vi "CTRE_Phoenix_CANifier_SetControlFramePeriod.vi"(8 "error in (no error)":errorcluster, 9 "periodMs":i32, 10 "Control Frame":T2=50593792 items=["Control_1_General"=50593792, "Control_2_PwmOutput"=50593856], 11 "CANifierDevRef":T1) -> (0 "error out":errorcluster, 3 "CANifierDevRef":T1)   [LabVIEW 2017]
doc: "Set the period of the specified control frame."
uses:
  CTRE_CANifier_DeviceRef.ctl
  CTRE_CANifier_ControlFrame.ctl
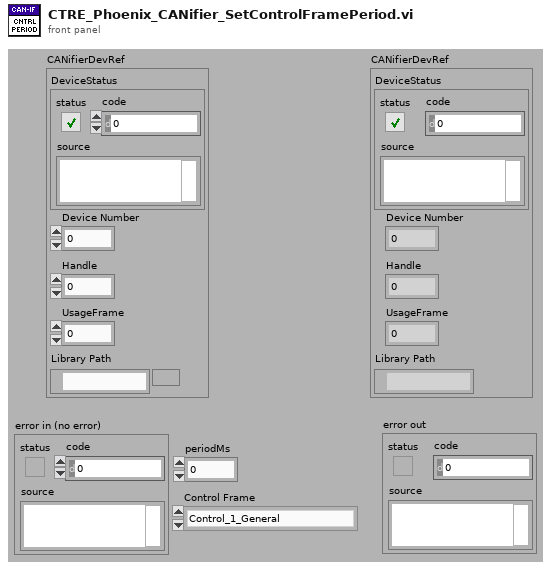
[diagram p1: front panel]
types:
  T1 = typedef "CTRE_CANifier_DeviceRef.ctl" = cluster{"DeviceStatus":errorcluster, "Device Number":u8, "Handle":u64, "UsageFrame":u32, "Library Path":path}
  T2 = typedef "CTRE_CANifier_ControlFrame.ctl" = u32
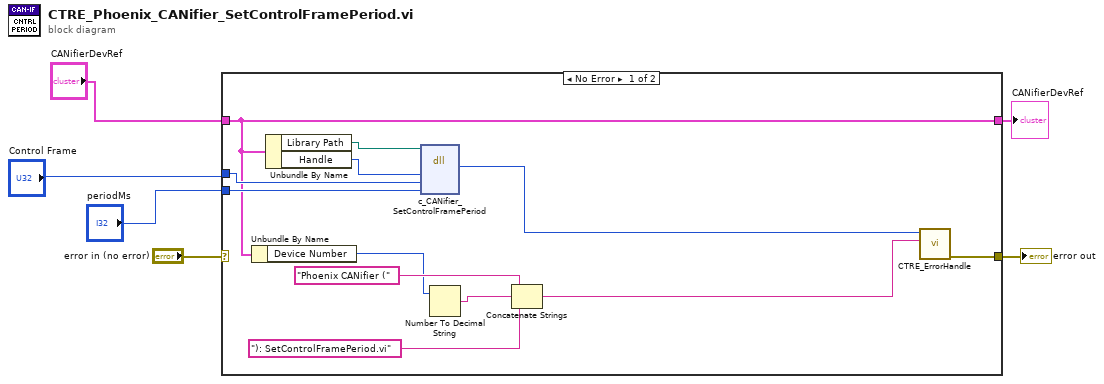
[diagram p0: block diagram]
diagram:
  n1 = case shown="No Error" "error in (no error)" {
    selector: "error in (no error)" -> [_ w20]
    tunnel: [w15 w20] -> w6
    tunnel: "CANifierDevRef" -> [w9 w19]
    tunnel: [w9 w19] -> w1
    tunnel: "Control Frame" -> [w12 _]
    tunnel: "periodMs" -> [w11 _]
    frame No Error {
      n2 = Unbundle By Name(w9) -> ("Device Number"=w10:u8)
      n3 = Unbundle By Name(w9) -> ("Library Path"=w8:path, "Handle"=w7:u64)
      n4 = dll-call lib="?" fn="c_CANifier_SetControlFramePeriod"(path in=w8, "handle"=w7, "frame"=w12, "periodMs"=w11) -> ("ErrorCode"=w13:i32)  [unwired: 5 in, 2 out]
      n5 = Number To Decimal String(number=w10) -> (decimal integer string=w17:string)  [unwired: 1 in]
      n6 = Concatenate Strings("Phoenix CANifier (" ("string"), w17, "): SetControlFramePeriod.vi" ("string")) -> (w14:string)
      n7 = call "CTRE_ErrorHandle.vi"("origin"=w14, "code"=w13) -> ("error out"=w15:errorcluster)  [unwired: 9 in]
    }
    frame Error {
    }
  }
  "error out" <- w6
  "CANifierDevRef" <- w1
